vi "dotNETDataTableTo2dArray.vi"(8 "error in (no error)":errorcluster caption="Fehler (Eingang, kein Fehler)", 10 "myDataTable":refnum<k24>, 11 "LoadConfigurationDataBase Eingang":refnum<class "LoadConfigurationDataBase.lvclass"> caption="DNL_LabVIEW Object in") -> (0 "error out":errorcluster caption="Fehler (Ausgang)", 2 "Array":string[][](array[string]), 3 "LoadConfigurationDataBase Ausgang":refnum<class "LoadConfigurationDataBase.lvclass"> caption="DNL_LabVIEW Object out")   [LabVIEW 2013, in "LoadConfigurationDataBase.lvclass"]
uses:
  LoadConfigurationDataBase.lvclass
  System.Data
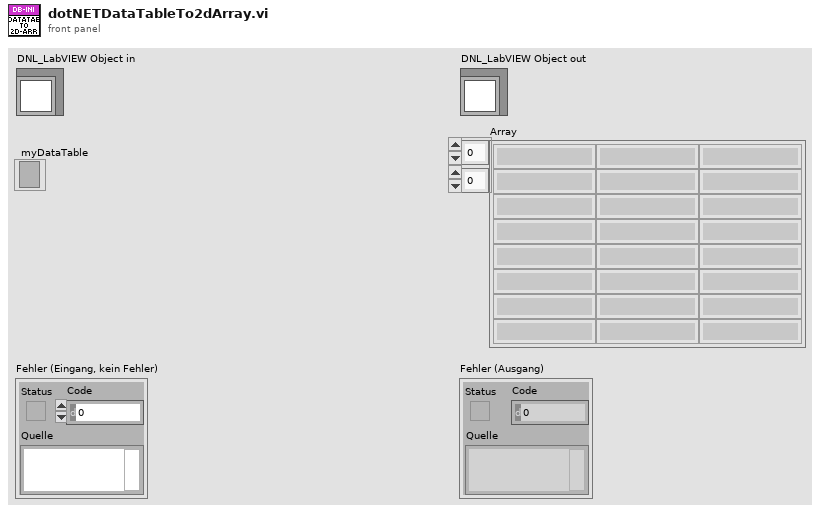
[diagram p1: front panel]
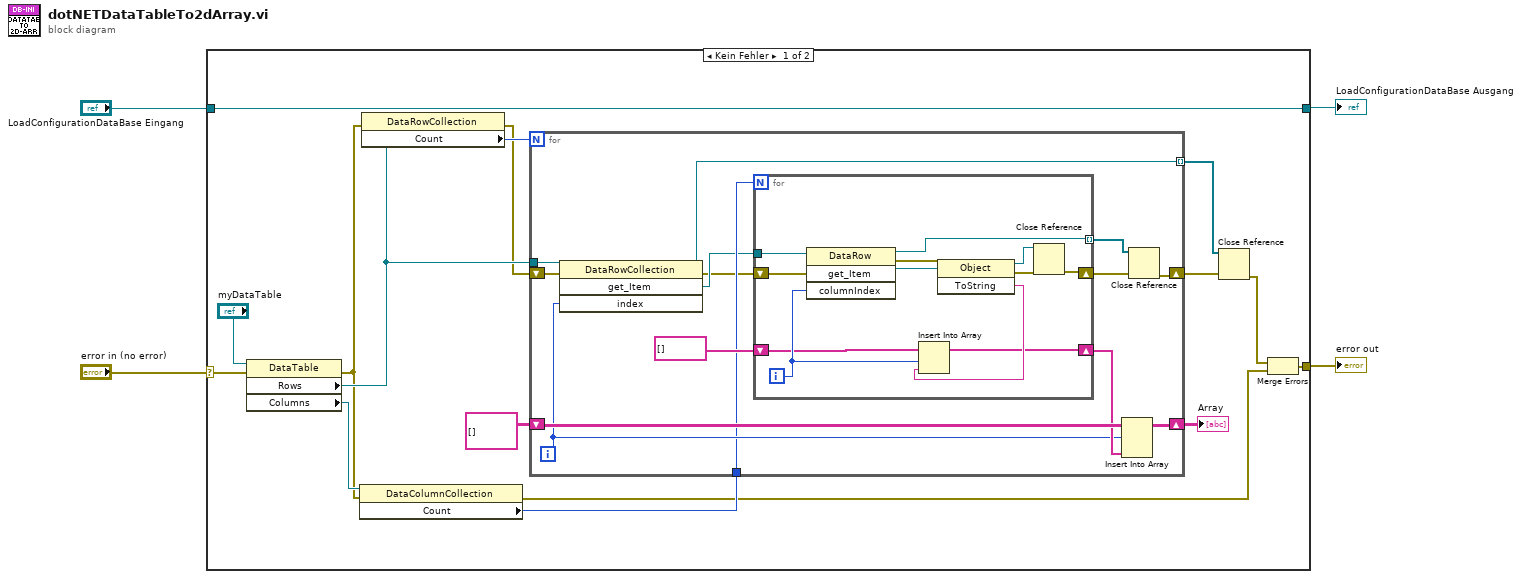
[diagram p0: block diagram]
diagram:
  n1 = case shown="Kein Fehler" "error in (no error)" {
    selector: "error in (no error)" -> [w12 w48]
    tunnel: [w7 w48] -> w3
    tunnel: [w20 w47] -> w1
    tunnel: "LoadConfigurationDataBase Eingang" -> [w20 w47]
    frame No Error {
      n2 = property class="DataTable"(reference="myDataTable", error in=w12) -> (error out=w11:errorcluster, "Rows"=w17:refnum<k24>, "Columns"=w19:refnum<k24>)  [unwired: 1 out]
      n3 = property class="DataColumnCollection"(reference=w19, error in=w11) -> (error out=w6:errorcluster, "Count"=w15:i32)  [unwired: 1 out]
      n4 = property class="DataRowCollection"(reference=w17, error in=w11) -> (error out=w10:errorcluster, "Count"=w18:i32)  [unwired: 1 out]
      n5 = for {
        N: w18 -> [_]
        tunnel: w17 -> [w34]
        shift-right: [w33] -> w14
        shift-left: string[][] [] -> [w32]
        tunnel: w15 -> [w28]
        shift-right: [w24] -> w9
        shift-left: w10 -> [w26]
        tunnel: [w21] -> w8 mode=indexing
        i -> [w29]
        n6 = invoke class="DataRowCollection" method="get_Item"(reference=w34, error in=w26, "index"=w29) -> (reference out=w21:refnum<k24>, error out=w25:errorcluster, "get_Item"=w27:refnum<k24>)  [unwired: 1 in, 1 out]
        n7 = for {
          N: w28 -> [_]
          shift-right: [w41] -> w30
          shift-left: string[] [] -> [w42]
          tunnel: w27 -> [w46]
          shift-right: [w38] -> w23
          shift-left: w25 -> [w40]
          tunnel: [w35] -> w22 mode=indexing
          i -> [w45]
          n8 = invoke class="DataRow" method="get_Item"(reference=w46, error in=w40, "columnIndex"=w45) -> (reference out=w35:refnum<k24>, error out=w39:errorcluster, "get_Item"=w44:refnum<k24>)  [unwired: 1 in, 1 out]
          n9 = invoke class="Object" method="ToString"(reference=w44, error in=w39) -> (reference out=w36:refnum<k24>, error out=w37:errorcluster, "ToString"=w43:string)  [unwired: 1 in]
          n10 = Insert Into Array(array=w42, index=w45, new element=w43) -> (w41:string[])
          n11 = Close Reference(reference=w36, error in (no error)=w37) -> (error out=w38:errorcluster)
        }
        n12 = Insert Into Array(array=w32, index (row)=w29, new element=w30) -> (w33:string[][])  [unwired: 1 in]
        n13 = Close Reference(reference=w22, error in (no error)=w23) -> (error out=w24:errorcluster)
      }
      "Array" <- w14
      n14 = Close Reference(reference=w8, error in (no error)=w9) -> (error out=w5:errorcluster)
      n15 = Merge Errors(w5, w6) -> (w7:errorcluster)
    }
    frame Error {
    }
  }
  "error out" <- w3
  "LoadConfigurationDataBase Ausgang" <- w1
